vi "Palette Draw.vi"(9 "Show Grid?":bool, 10 "Include Palette Icon?":bool, 11 "Palettes":T2(array[cluster])) -> (2 "Palette Image":picture[](array[picture]), 3 "Palette Names":string[](array[string]))   [LabVIEW 2018, in "Markdown.lvlib"]
doc: "Draw diagram palette images as \"text and image\"."
uses:
  Markdown.lvlib
  TypeDefs/Item.ctl
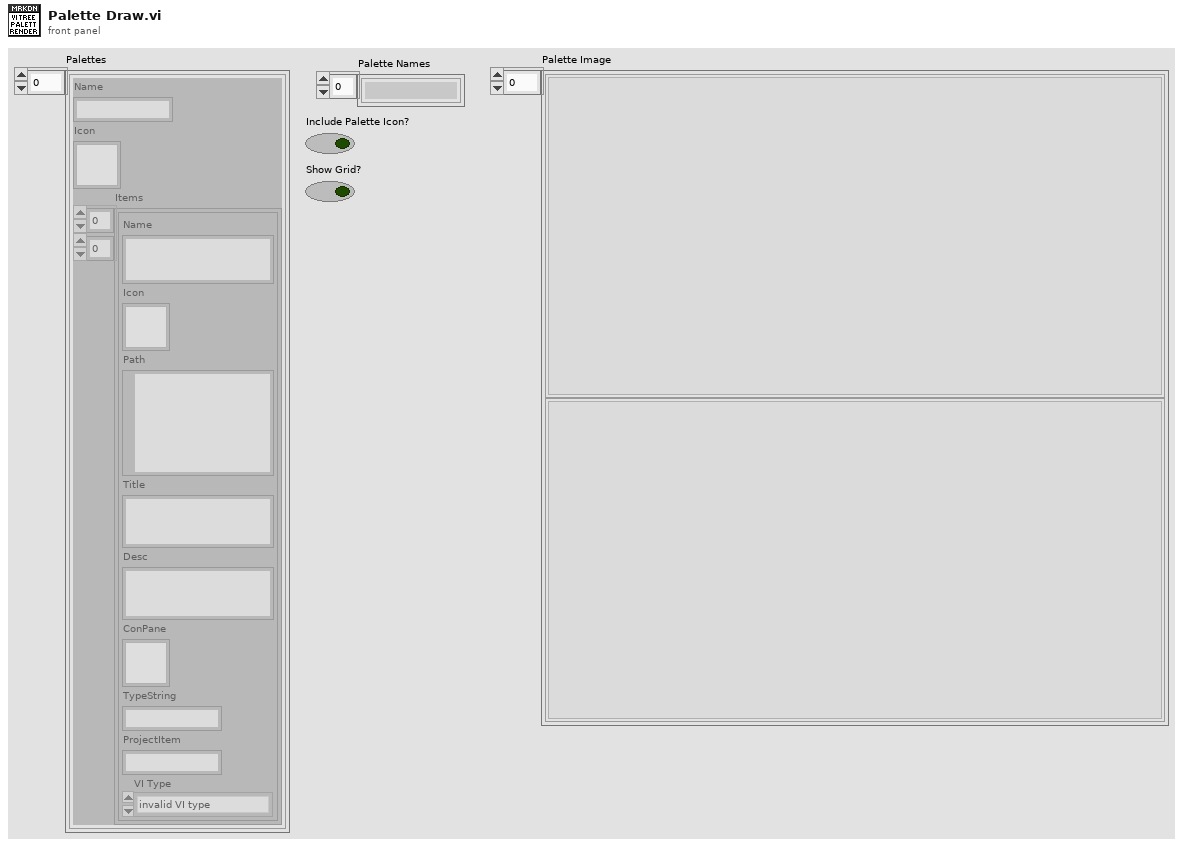
[diagram p1: front panel]
types:
  T1 = typedef "Markdown.lvlib/Item.ctl" = cluster{"Name":string, "Icon":picture, "Path":path, "Title":string, "Desc":string, "ConPane":picture, "TypeString":string, "ProjectItem":string, "VI Type":enum32{"invalid VI type", "Standard VI", "Control VI", "Global VI", "Polymorphic VI", "Configuration VI", "SubSystem", "Facade VI", "Method VI", "Statechart Diagram VI"}}
  T2 = cluster{"Name":string, "Icon":picture, "Items":T1[][]}[]
  T3 = cluster{"left":i16, "top":i16, "right":i16, "bottom":i16}
  T4 = cluster{"horizontal":enum16{"left", "center", "right"}, "vertical":enum16{"top", "center", "bottom"}}
  T5 = cluster{"Width":u16, "Style":enum32{"Solid", "Dash", "Dot", "DashDot", "DashDotDot"}}
  T6 = typedef "imagedata.ctl" = cluster{"image type":i32, "image depth":i32, "image":u8[], "mask":u8[], "colors":u32[], "Rectangle":cluster{"left":i16, "top":i16, "right":i16, "bottom":i16}}
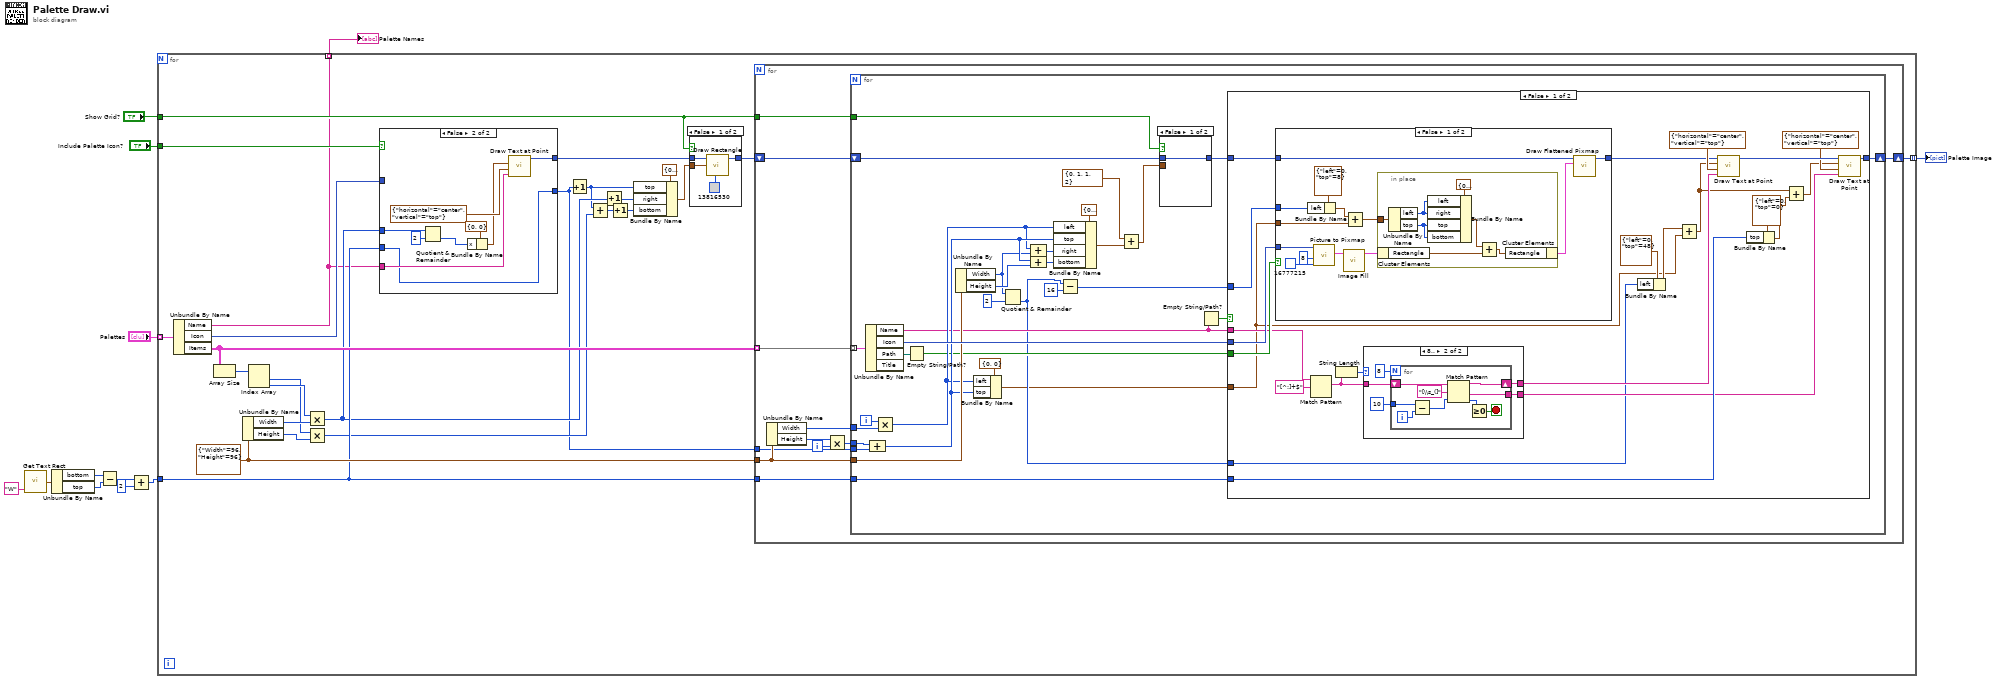
[diagram p0: block diagram]
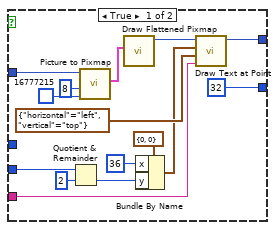
[diagram p3: hidden frame]
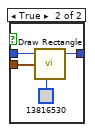
[diagram p4: hidden frame]
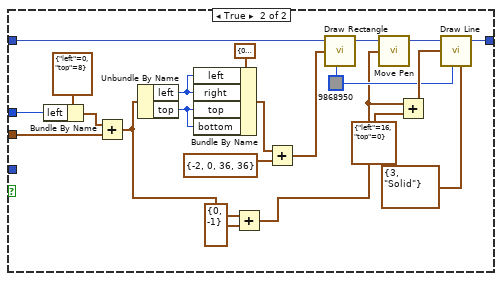
[diagram p5: hidden frame]
diagram:
  n1 = call <vilib>:"Get Text Rect.vi"("text"="W") -> ("rect"=w9:T3)  [unwired: 8 in]
  n2 = Unbundle By Name(w9) -> ("bottom"=w8:i16, "top"=w7:i16)
  n3 = Subtract(x=w8, y=w7) -> (x-y=w6:i16)
  n4 = Add(x=w6, y=i16 2) -> (x+y=w5:i16)
  n5 = for {
    tunnel: "Palettes" -> [w37] mode=indexing
    tunnel: [w36] -> w11 mode=indexing
    tunnel: w5 -> [w29]
    tunnel: "Include Palette Icon?" -> [w28]
    tunnel: "Show Grid?" -> [w25]
    tunnel: [w13] -> w1 mode=indexing
    w33 = cluster{"Width":i32, "Height":i32} {"Width"=96, "Height"=96} ("x")
    n6 = Unbundle By Name(w37) -> ("Name"=w13:string, "Icon"=w30:picture, "Items"=w35:T1[][])
    n7 = Array Size(array=w35) -> (size(s)=w34:i32[])
    n8 = Unbundle By Name(w33) -> ("Width"=w32:i32, "Height"=w21:i32)
    n9 = Index Array(array=w34) -> (element #1=w20:i32, element #2=w31:i32)  [unwired: 2 in]
    n10 = Multiply(x=w31, y=w32) -> (x*y=w22:i32)
    n11 = Multiply(x=w20, y=w21) -> (x*y=w19:i32)
    n12 = case shown="False" w28 {
      tunnel: [w55 w64] -> w27
      tunnel: [i16 32 w60] -> w17
      tunnel: w30 -> [w49 _]
      tunnel: w29 -> [w45 w60]
      tunnel: w13 -> [w43 w61]
      tunnel: w22 -> [_ w59]
      frame True {
        n13 = Quotient & Remainder(x=w45, y=2) -> (floor(x/y)=w44:i32)  [unwired: 1 out]
        n14 = call <vilib>:"Picture to Pixmap.vi"("Background Color"=u32 16777215, "depth"=8, "picture"=w49) -> ("image data"=w48:T6)  [unwired: 7 in, 1 out]
        n15 = call <vilib>:"Draw Flattened Pixmap.vi"("image data"=w48) -> ("new picture"=w47:picture)  [unwired: 8 in]
        n16 = Bundle By Name(cluster=cluster{"x":i16, "y":i16} {"x"=0, "y"=0} ("origin"), "x"=i16 36, "y"=w44) -> (w53:cluster{"x":i16, "y":i16})
        n17 = call <vilib>:"Draw Text at Point.vi"("text"=w43, "alignment(left, top)"=T4 {"horizontal"=enum."left", "vertical"=enum."top"}, "origin"=w53, "picture"=w47) -> ("new picture"=w55:picture)  [unwired: 6 in, 1 out]
      }
      frame False {
        n18 = Quotient & Remainder(x=w59, y=2) -> (floor(x/y)=w58:i32)  [unwired: 1 out]
        n19 = Bundle By Name(cluster=cluster{"x":i16, "y":i16} {"x"=0, "y"=0} ("origin"), "x"=w58) -> (w62:cluster{"x":i16, "y":i16})
        n20 = call <vilib>:"Draw Text at Point.vi"("text"=w61, "alignment(left, top)"=T4 {"horizontal"=enum."center", "vertical"=enum."top"}, "origin"=w62) -> ("new picture"=w64:picture)  [unwired: 7 in, 1 out]
      }
    }
    n21 = Increment(x=w17) -> (x+1=w16:i16)
    n22 = Add(x=w16, y=w19) -> (x+y=w18:i32)
    n23 = Increment(x=w22) -> (x+1=w14:i32)
    n24 = Increment(x=w18) -> (x+1=w15:i32)
    n25 = Bundle By Name(cluster=T3 {"left"=0, "top"=0, "right"=0, "bottom"=0}, "top"=w16, "right"=w14, "bottom"=w15) -> (w23:T3)
    n26 = case shown="False" w25 {
      tunnel: w27 -> [w41 w42]
      tunnel: [w40 w42] -> w26
      tunnel: w23 -> [w38 _]
      frame False {
        n27 = call <vilib>:"Draw Rectangle.vi"("picture"=w41, "rect"=w38, "color(black)"=u32 13816530) -> ("new picture"=w40:picture)  [unwired: 6 in]
      }
      frame True {
      }
    }
    n28 = for {
      tunnel: w35 -> [w77] mode=indexing
      shift-right: [w76] -> w36
      shift-left: w26 -> [w75]
      tunnel: w33 -> [w70]
      tunnel: w29 -> [w69]
      tunnel: w17 -> [w68]
      tunnel: w25 -> [w67]
      i -> [w73]
      n29 = Unbundle By Name(w70) -> ("Width"=w71:i32, "Height"=w74:i32)
      n30 = Multiply(x=w74, y=w73) -> (x*y=w72:i32)
      n31 = for {
        tunnel: w77 -> [w109] mode=indexing
        shift-right: [w103] -> w76
        shift-left: w75 -> [w107]
        tunnel: w72 -> [w105]
        tunnel: w71 -> [w104]
        tunnel: w70 -> [w101]
        tunnel: w69 -> [w102]
        tunnel: w68 -> [w100]
        tunnel: w67 -> [w78]
        i -> [w106]
        n32 = Unbundle By Name(w109) -> ("Name"=w95:string, "Icon"=w108:picture, "Path"=w97:path)  [unwired: 1 out]
        n33 = Compound Arithmetic op=unknown(w105, w100) -> (w99:i32)
        n34 = Multiply(x=w106, y=w104) -> (x*y=w98:i32)
        n35 = Empty String/Path?(string/path=w97) -> (empty?=w96:bool)
        n36 = Unbundle By Name(w101) -> ("Width"=w86:i32, "Height"=w88:i32)
        n37 = Bundle By Name(cluster=cluster{"left":i16, "top":i16} {"left"=0, "top"=0} ("x"), "left"=w98, "top"=w99) -> (w80:cluster{"left":i16, "top":i16})
        n38 = Quotient & Remainder(x=w86, y=2) -> (floor(x/y)=w94:i32)  [unwired: 1 out]
        n39 = Compound Arithmetic op=ADD(w98, w86) -> (w89:i32)
        n40 = Compound Arithmetic op=unknown(w99, w88) -> (w90:i32)
        n41 = Bundle By Name(cluster=T3 {"left"=0, "top"=0, "right"=0, "bottom"=0} ("rect"), "left"=w98, "top"=w99, "right"=w89, "bottom"=w90) -> (w91:T3)
        n42 = Subtract(x=w94, y=16) -> (x-y=w85:i32)
        n43 = Add(x=T3 {"left"=0, "top"=1, "right"=1, "bottom"=2} ("rect"), y=w91) -> (x+y=w83:T3)
        n44 = case shown="False" w78 {
          tunnel: w107 -> [w110 w114]
          tunnel: [w110 w113] -> w93
          tunnel: w83 -> [_ w111]
          frame False {
          }
          frame True {
            n45 = call <vilib>:"Draw Rectangle.vi"("picture"=w114, "rect"=w111, "color(black)"=u32 13816530) -> ("new picture"=w113:picture)  [unwired: 6 in]
          }
        }
        n46 = Empty String/Path?(string/path=w95) -> (empty?=w79:bool)
        n47 = case shown="False" w79 {
          tunnel: w108 -> [w138 _]
          tunnel: [w137 w195] -> w103
          tunnel: w102 -> [w136 _]
          tunnel: w96 -> [w135 _]
          tunnel: w95 -> [w134 _]
          tunnel: w94 -> [w118 _]
          tunnel: w93 -> [w117 w195]
          tunnel: w85 -> [w116 _]
          tunnel: w80 -> [w115 _]
          frame False {
            n48 = case shown="False" w135 {
              tunnel: w138 -> [w151 _]
              tunnel: [w150 w166] -> w132
              tunnel: w117 -> [w149 w179]
              tunnel: w116 -> [w148 w170]
              tunnel: w115 -> [w141 w169]
              frame False {
                n49 = Bundle By Name(cluster=cluster{"left":i16, "top":i16} {"left"=0, "top"=8} ("x"), "left"=w148) -> (w142:cluster{"left":i16, "top":i16})
                n50 = call <vilib>:"Picture to Pixmap.vi"("Background Color"=u32 16777215, "depth"=8, "picture"=w151) -> ("image data"=w140:T6)  [unwired: 7 in, 1 out]
                n51 = call "Image Fill.vi"("image data in"=w140) -> ("image data out"=w139:T6)  [unwired: 10 in]
                n52 = Add(x=w142, y=w141) -> (x+y=w144:cluster{"left":i16, "top":i16})
                n53 = in-place {
                  in-place-border: w144 -> [w154]
                  n54 = in-place-cluster #1(w139) -> ("Rectangle"=w158:T3)
                  n55 = Unbundle By Name(w154) -> ("left"=w153:i16, "top"=w152:i16)
                  n56 = Bundle By Name(cluster=T3 {"left"=0, "top"=0, "right"=0, "bottom"=0} ("x"), "left"=w153, "right"=w153, "top"=w152, "bottom"=w152) -> (w155:T3)
                  n57 = Add(x=w155, y=w158) -> (x+y=w156:T3)
                  n58 = in-place-cluster #1("Rectangle"=w156) -> (w145:T6)
                }
                n59 = call <vilib>:"Draw Flattened Pixmap.vi"("image data"=w145, "picture"=w149) -> ("new picture"=w150:picture)  [unwired: 7 in]
              }
              frame True {
                w163 = u32 9868950 ("color(black)")
                n60 = Bundle By Name(cluster=cluster{"left":i16, "top":i16} {"left"=0, "top"=8} ("x"), "left"=w170) -> (w171:cluster{"left":i16, "top":i16})
                n61 = Add(x=w171, y=w169) -> (x+y=w160:cluster{"left":i16, "top":i16})
                n62 = Unbundle By Name(w160) -> ("left"=w177:i16, "top"=w176:i16)
                n63 = Bundle By Name(cluster=T3 {"left"=0, "top"=0, "right"=0, "bottom"=0} ("x"), "left"=w177, "right"=w177, "top"=w176, "bottom"=w176) -> (w174:T3)
                n64 = Add(x=w160, y=cluster{"left":i16, "top":i16} {"left"=0, "top"=-1}) -> (x+y=w159:cluster{"left":i16, "top":i16})
                n65 = Add(x=w174, y=T3 {"left"=-2, "top"=0, "right"=36, "bottom"=36} ("x")) -> (x+y=w173:T3)
                n66 = call <vilib>:"Draw Rectangle.vi"("picture"=w179, "rect"=w173, "color(black)"=w163) -> ("new picture"=w167:picture)  [unwired: 6 in]
                n67 = call <vilib>:"Move Pen.vi"("new position"=w159, "picture"=w167) -> ("new picture"=w168:picture)  [unwired: 3 in]
                n68 = Add(x=w159, y=cluster{"left":i16, "top":i16} {"left"=16, "top"=0} ("x")) -> (x+y=w164:cluster{"left":i16, "top":i16})
                n69 = call <vilib>:"Draw Line.vi"("picture"=w168, "end point"=w164, "color(black)"=w163, "pen"=T5 {"Width"=3, "Style"=enum."Solid"}) -> ("new picture"=w166:picture)  [unwired: 5 in]
              }
            }
            n70 = Match Pattern(string=w134, regular expression="[^:]+$") -> (match substring=w121:string)  [unwired: 1 in, 3 out]
            n71 = String Length(string=w121) -> (length=w120:i32)
            n72 = case shown="8.." w120 {
              tunnel: [w180 w183] -> w130
              tunnel: [_ w182] -> w127
              tunnel: w121 -> [w180 w184]
              frame ..7 {
              }
              frame 8.. {
                n73 = for {
                  N: 8 -> [_]
                  tunnel: 10 ("offset (0)") -> [w193]
                  tunnel: [w190] -> w182
                  shift-right: [w191] -> w183
                  shift-left: w184 -> [w192]
                  i -> [w188]
                  stop <- w186 stop-if-true
                  n74 = Subtract(x=w193, y=w188) -> (x-y=w189:i32)
                  n75 = Match Pattern(string=w192, regular expression="[\\s_(]", offset (0)=w189) -> (before substring=w191:string, after substring=w190:string, offset past match=w187:i32)  [unwired: 1 out]
                  n76 = Greater Or Equal To 0?(x=w187) -> (x >= 0?=w186:bool)
                }
              }
            }
            n77 = Bundle By Name(cluster=cluster{"left":i16, "top":i16} {"left"=0, "top"=48} ("x"), "left"=w118) -> (w119:cluster{"left":i16, "top":i16})
            n78 = Add(x=w119, y=w115) -> (x+y=w122:cluster{"left":i16, "top":i16})
            n79 = call <vilib>:"Draw Text at Point.vi"("text"=w130, "alignment(left, top)"=T4 {"horizontal"=enum."center", "vertical"=enum."top"}, "origin"=w122, "picture"=w132) -> ("new picture"=w129:picture)  [unwired: 6 in, 1 out]
            n80 = Bundle By Name(cluster=cluster{"left":i16, "top":i16} {"left"=0, "top"=0} ("x"), "top"=w136) -> (w125:cluster{"left":i16, "top":i16})
            n81 = Add(x=w122, y=w125) -> (x+y=w124:cluster{"left":i16, "top":i16})
            n82 = call <vilib>:"Draw Text at Point.vi"("text"=w127, "alignment(left, top)"=T4 {"horizontal"=enum."center", "vertical"=enum."top"}, "origin"=w124, "picture"=w129) -> ("new picture"=w137:picture)  [unwired: 6 in, 1 out]
          }
          frame True {
          }
        }
      }
    }
  }
  "Palette Image" <- w11
  "Palette Names" <- w1
